vi "Generate Results.vi"(8 "error in (no error)":errorcluster) -> (0 "error out":errorcluster, 3 "Data":T1[](array[typedef])=[{"Name"="Test Case.lvclass:Test Failing Test.vi", "Message"="Message", "Description"="Description", "Status"=enum."Failed", "Result Type"=enum."Fail", "Execution Time"=0.0}, {"Name"="Test Case.lvclass:Test Failing Test.vi", "Message"="", "Description"="Failed:\nDescription\nMessage", "Status"=enum."Failed", "Result Type"=enum."Test Case", "Execution Time"=0.013}, {"Name"="Test Case.lvclass:Test Passing Test.vi", "Message"="Message", "Description"="Description", "Status"=enum."Passed", "Result Type"=enum."Pass", "Execution Time"=0.0}, {"Name"="Test Case.lvclass:Test Passing Test.vi", "Message"="", "Description"="Passed:\nDescription\nMessage", "Status"=enum."Passed", "Result Type"=enum."Test Case", "Execution Time"=0.022}, {"Name"="Test Case.lvclass", "Message"="", "Description"="", "Status"=enum."Failed", "Result Type"=enum."Test Suite", "Execution Time"=0.0}, {"Name"="Test Suite", "Message"="", "Description"="", "Status"=enum."Failed", "Result Type"=enum."Test Suite", "Execution Time"=0.0}])   [LabVIEW 2020, in "XML Report Test.lvclass"]
uses:
  XML Report Test.lvclass
  source/Core/Result/Result.ctl
  source/Core/Result/Status.ctl
  source/Core/Result/Type.ctl
  XML Report Test.lvclass/XML Report Test.ctl
  source/Core/Result/Result.lvlib
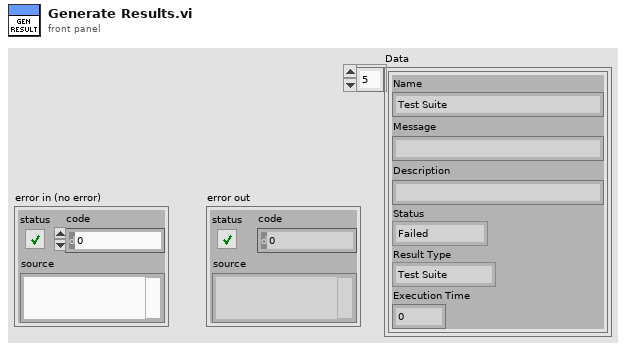
[diagram p1: front panel]
types:
  T1 = typedef "Result.lvlib/Result.ctl" = cluster{"Name":string, "Message":string, "Description":string, "Status":T2, "Result Type":T3, "Execution Time":dbl}
  T2 = typedef "Result.lvlib/Status.ctl" = enum16{"", "Passed", "Failed", "Error", "Skipped", "Setup Error", "Broken", "Teardown Error"}
  T3 = typedef "Result.lvlib/Type.ctl" = enum16{"Test Case", "Test Suite", "Test Run", "Pass", "Fail", "Skip", "Pass if", "Fail if", "Pass if Error", "Fail if Error", "Pass if Equal", "Fail if Equal"}
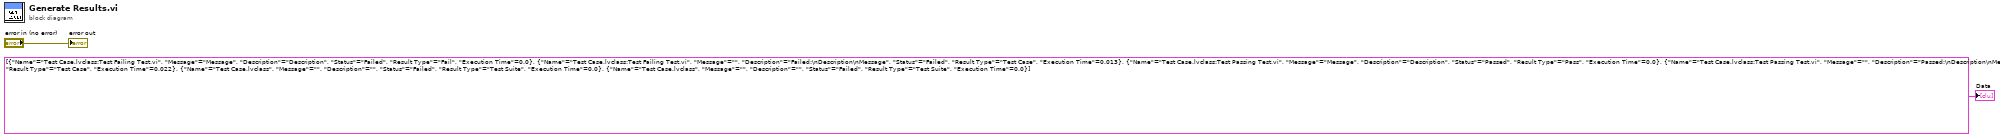
[diagram p0: block diagram]
diagram:
  "error out" <- "error in (no error)"
  "Data" <- T1[] [{"Name"="Test Case.lvclass:Test Failing Test.vi", "Message"="Message", "Description"="Description", "Status"=enum."Failed", "Result Type"=enum."Fail", "Execution Time"=0.0}, {"Name"="Test Case.lvclass:Test Failing Test.vi", "Message"="", "Description"="Failed:\nDescription\nMessage", "Status"=enum."Failed", "Result Type"=enum."Test Case", "Execution Time"=0.013}, {"Name"="Test Case.lvclass:Test Passing Test.vi", "Message"="Message", "Description"="Description", "Status"=enum."Passed", "Result Type"=enum."Pass", "Execution Time"=0.0}, {"Name"="Test Case.lvclass:Test Passing Test.vi", "Message"="", "Description"="Passed:\nDescription\nMessage", "Status"=enum."Passed", "Result Type"=enum."Test Case", "Execution Time"=0.022}, {"Name"="Test Case.lvclass", "Message"="", "Description"="", "Status"=enum."Failed", "Result Type"=enum."Test Suite", "Execution Time"=0.0}, {"Name"="Test Case.lvclass", "Message"="", "Description"="", "Status"=enum."Failed", "Result Type"=enum."Test Suite", "Execution Time"=0.0}] ("Array")
